vi "U32toRgba_2D.vi"(11 "U32":u32[][](array[numeric])) -> (3 "Rgba":T1[][](array[typedef]))   [LabVIEW 2024, in "OpenLvVision_Image.lvlib" / "DataAccess.lvlib"]
doc: "Convert an number into an cluster"
uses:
  DataAccess.lvlib
  TypeDef/RgbaU32.ctl
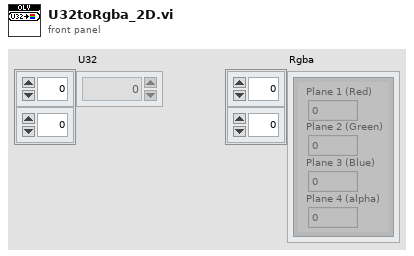
[diagram p1: front panel]
types:
  T1 = typedef "OpenLvVision_Image.lvlib/DataAccess.lvlib/RgbaU32.ctl" = cluster{"Plane 1 (Red)":u8, "Plane 2 (Green)":u8, "Plane 3 (Blue)":u8, "Plane 4 (alpha)":u8}
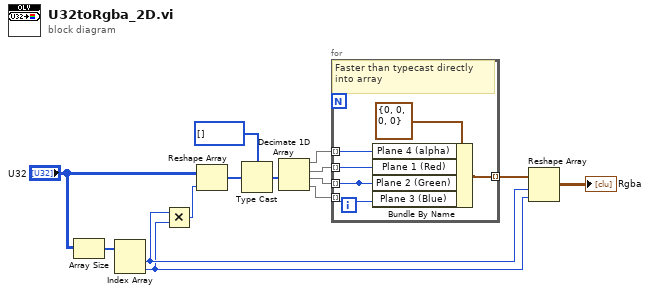
[diagram p0: block diagram]
diagram:
  n1 = Array Size(array="U32") -> (size(s)=w8:i32[])
  n2 = Index Array(array=w8) -> (element #1=w3:i32, element #2=w1:i32)  [unwired: 2 in]
  n3 = Multiply(x=w3, y=w1) -> (x*y=w2:i32)
  n4 = Reshape Array("U32", w2) -> (w4:u32[])
  n5 = Type Cast(type=u8[] [], x=w4) -> (*(type *) &x=w13:u8[])
  n6 = Decimate 1D Array(w13) -> (w12:u8[], w10:u8[], w9:u8[], w11:u8[])
  n7 = for {
    tunnel: w12 -> [w20] mode=indexing
    tunnel: w10 -> [w19] mode=indexing
    tunnel: [w15] -> _ mode=indexing
    tunnel: w11 -> [w18] mode=indexing
    tunnel: [w17] -> w7 mode=indexing
    tunnel: w9 -> [w15] mode=indexing
    # "Faster than typecast directly into array"
    n8 = Bundle By Name(cluster=T1 {"Plane 1 (Red)"=0, "Plane 2 (Green)"=0, "Plane 3 (Blue)"=0, "Plane 4 (alpha)"=0} ("Color"), "Plane 4 (alpha)"=w20, "Plane 1 (Red)"=w19, "Plane 2 (Green)"=w15, "Plane 3 (Blue)"=w18) -> (w17:T1)
  }
  n9 = Reshape Array(w7, w3, w1) -> (→"Rgba":T1[][])
